vi "Build Sweep Measurements Results.vi"(8 "measurement results in":T2 {"Gain" format="%_6g"; "THD" format="%_6g"; "THD+N" format="%_6g"; "SNR" format="%_6g"; "SFDR (dBc)" format="%_6g"; "Dynamic range (dB)" format="%_6g"; "Phase (deg)" format="%_6g"; "Amplitude (dB)" format="%_6g"; "Amplitude (V)" format="%_6g"; "Frequency (Hz)" format="%_6g"; "df" format="%_6g"; "f0" format="%_6g"; "dt" format="%_6g"; "Frequency domain" format="%_6g"; "Time domain" format="%_6g"}, 9 "spectra":cluster{"x0":dbl, "dx":dbl, "magnitude":dbl[]}[](array[cluster]), 10 "waveforms":waveform(dbl)[](array[waveform]), 11 "results":T1(array[cluster])) -> (0 "measurement results out":T2 {"Gain" format="%_6g"; "THD" format="%_6g"; "THD+N" format="%_6g"; "SNR" format="%_6g"; "SFDR (dBc)" format="%_6g"; "Dynamic range (dB)" format="%_6g"; "Phase (deg)" format="%_6g"; "Amplitude (dB)" format="%_6g"; "Amplitude (V)" format="%_6g"; "Frequency (Hz)" format="%_6g"; "df" format="%_6g"; "f0" format="%_6g"; "dt" format="%_6g"; "Frequency domain" format="%_6g"; "Time domain" format="%_6g"})   [LabVIEW 2021, in "Stepped Frequency Sweep_Audio DAC.lvlib"]
uses:
  Measurement Results.ctl
  Stepped Frequency Sweep_Audio DAC.lvlib
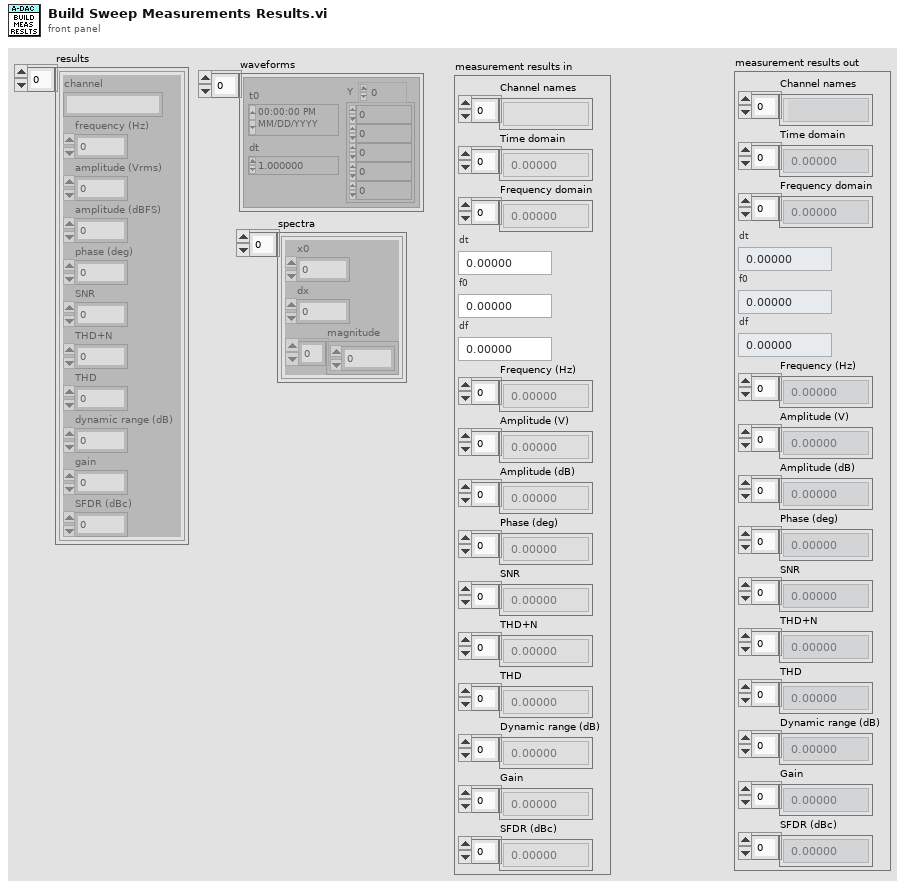
[diagram p1: front panel]
types:
  T1 = cluster{"channel":string, "frequency (Hz)":dbl, "amplitude (Vrms)":dbl, "amplitude (dBFS)":dbl, "phase (deg)":dbl, "SNR":dbl, "THD+N":dbl, "THD":dbl, "dynamic range (dB)":dbl, "gain":dbl, "SFDR (dBc)":dbl}[]
  T2 = typedef "Stepped Frequency Sweep_Audio DAC.lvlib/Measurement Results.ctl" = cluster{"Channel names":string[], "Time domain":dbl[], "Frequency domain":dbl[], "dt":dbl, "f0":dbl, "df":dbl, "Frequency (Hz)":dbl[], "Amplitude (V)":dbl[], "Amplitude (dB)":dbl[], "Phase (deg)":dbl[], "SNR":dbl[], "THD+N":dbl[], "THD":dbl[], "Dynamic range (dB)":dbl[], "Gain":dbl[], "SFDR (dBc)":dbl[]}
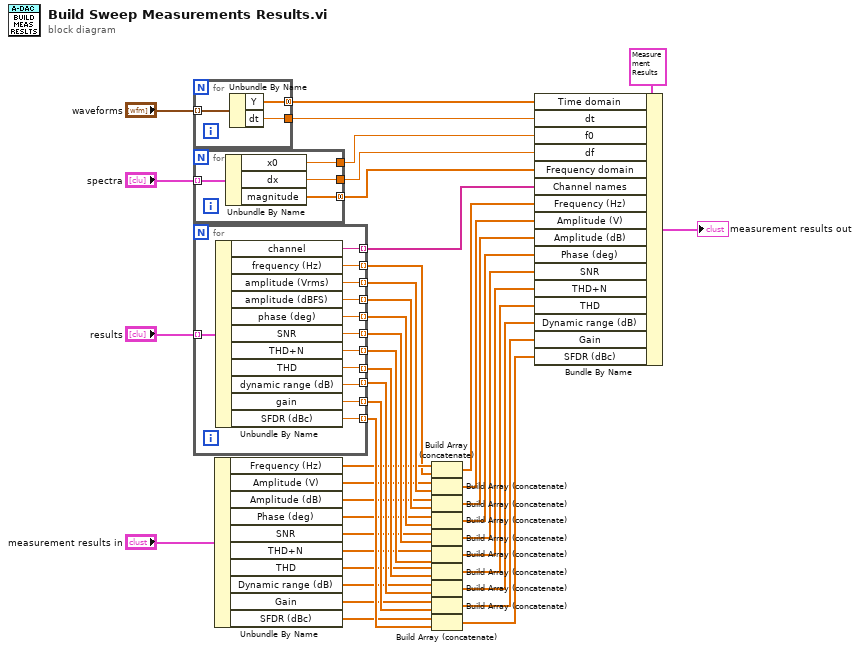
[diagram p0: block diagram]
diagram:
  n1 = for {
    tunnel: "waveforms" -> [w45] mode=indexing
    tunnel: [w44] -> w5 mode=concatenating
    tunnel: [w43] -> w4
    n2 = Unbundle By Name(w45) -> ("Y"=w44:dbl[], "dt"=w43:dbl)
  }
  n3 = for {
    tunnel: "spectra" -> [w49] mode=indexing
    tunnel: [w48] -> w3
    tunnel: [w47] -> w2
    tunnel: [w46] -> w1 mode=concatenating
    n4 = Unbundle By Name(w49) -> ("x0"=w48:dbl, "dx"=w47:dbl, "magnitude"=w46:dbl[])
  }
  n5 = for {
    tunnel: "results" -> [w61] mode=indexing
    tunnel: [w60] -> w42 mode=indexing
    tunnel: [w59] -> w11 mode=indexing
    tunnel: [w58] -> w24 mode=indexing
    tunnel: [w57] -> w25 mode=indexing
    tunnel: [w56] -> w26 mode=indexing
    tunnel: [w55] -> w27 mode=indexing
    tunnel: [w54] -> w28 mode=indexing
    tunnel: [w53] -> w29 mode=indexing
    tunnel: [w52] -> w30 mode=indexing
    tunnel: [w51] -> w31 mode=indexing
    tunnel: [w50] -> w32 mode=indexing
    n6 = Unbundle By Name(w61) -> ("channel"=w60:string, "frequency (Hz)"=w59:dbl, "amplitude (Vrms)"=w58:dbl, "amplitude (dBFS)"=w57:dbl, "phase (deg)"=w56:dbl, "SNR"=w55:dbl, "THD+N"=w54:dbl, "THD"=w53:dbl, "dynamic range (dB)"=w52:dbl, "gain"=w51:dbl, "SFDR (dBc)"=w50:dbl)
  }
  n7 = Unbundle By Name("measurement results in") -> ("Frequency (Hz)"=w13:dbl[], "Amplitude (V)"=w15:dbl[], "Amplitude (dB)"=w16:dbl[], "Phase (deg)"=w17:dbl[], "SNR"=w18:dbl[], "THD+N"=w19:dbl[], "THD"=w20:dbl[], "Dynamic range (dB)"=w21:dbl[], "Gain"=w22:dbl[], "SFDR (dBc)"=w23:dbl[])
  n8 = Build Array (concatenate)(w13, w11) -> (w14:dbl[])
  n9 = Build Array (concatenate)(w15, w24) -> (w33:dbl[])
  n10 = Build Array (concatenate)(w16, w25) -> (w34:dbl[])
  n11 = Build Array (concatenate)(w17, w26) -> (w35:dbl[])
  n12 = Build Array (concatenate)(w18, w27) -> (w36:dbl[])
  n13 = Build Array (concatenate)(w19, w28) -> (w37:dbl[])
  n14 = Build Array (concatenate)(w20, w29) -> (w38:dbl[])
  n15 = Build Array (concatenate)(w21, w30) -> (w39:dbl[])
  n16 = Build Array (concatenate)(w22, w31) -> (w40:dbl[])
  n17 = Build Array (concatenate)(w23, w32) -> (w41:dbl[])
  n18 = Bundle By Name(cluster=T2 {"Channel names"=[], "Time domain"=[], "Frequency domain"=[], "dt"=0.0, "f0"=0.0, "df"=0.0, "Frequency (Hz)"=[], "Amplitude (V)"=[], "Amplitude (dB)"=[], "Phase (deg)"=[], "SNR"=[], "THD+N"=[], "THD"=[], "Dynamic range (dB)"=[], "Gain"=[], "SFDR (dBc)"=[]} ("measurement results"), "Time domain"=w5, "dt"=w4, "f0"=w3, "df"=w2, "Frequency domain"=w1, "Channel names"=w42, "Frequency (Hz)"=w14, "Amplitude (V)"=w33, "Amplitude (dB)"=w34, "Phase (deg)"=w35, "SNR"=w36, "THD+N"=w37, "THD"=w38, "Dynamic range (dB)"=w39, "Gain"=w40, "SFDR (dBc)"=w41) -> (→"measurement results out":T2)
